vi "Send Command.vi"(8 "error in (no error)":errorcluster, 9 "Thread ID":u16, 10 "Message Queues":T3, 11 "Current Test":T1) -> (0 "error out":errorcluster)   [LabVIEW 2014]
uses:
  support/Message Queue/All Message Queues.ctl
  support/Message Queue/Message Cluster.ctl
  Teszt/Teszt.ctl
  Teszt/Command.ctl
  Message.ctl
  support/Message Queue/Enqueue Message (Single).vi
  support/Message Queue/Message Queue.lvlib
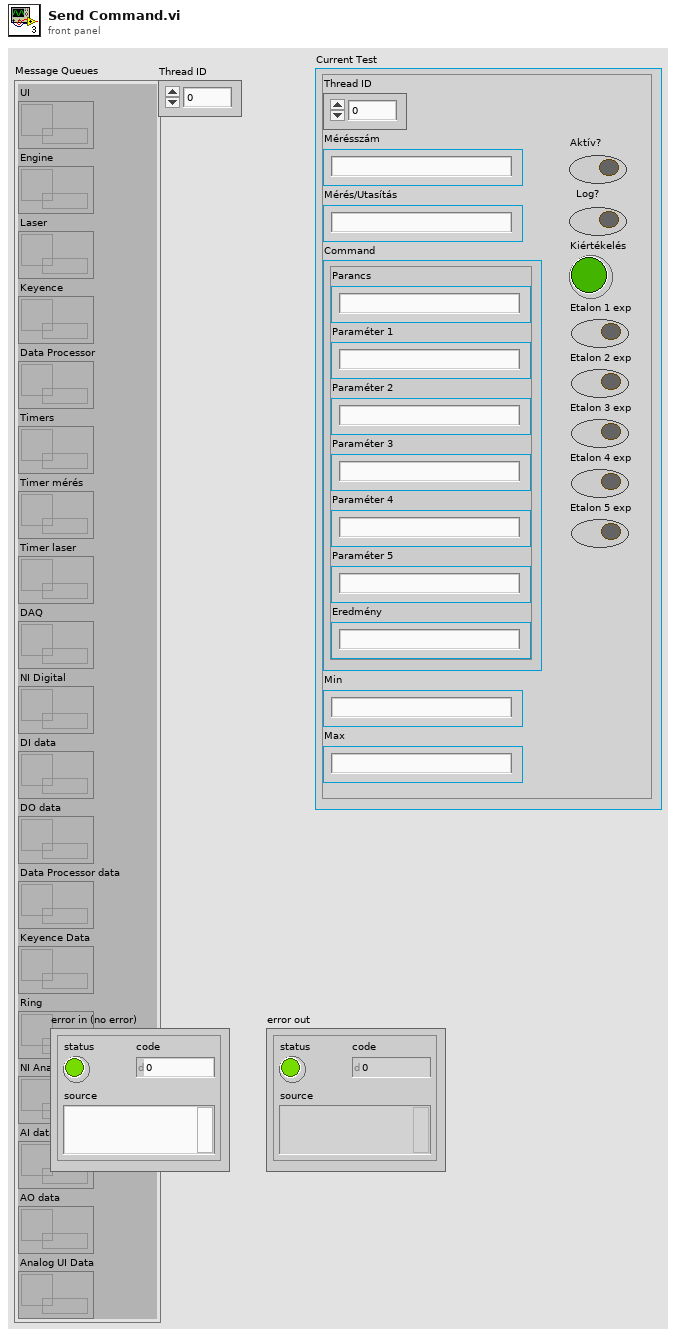
[diagram p1: front panel]
types:
  T1 = typedef "Teszt.ctl" = cluster{"Thread ID":dbl, "Mérésszám":string, "Mérés/Utasítás":string, "Command":T2, "Min":string, "Max":string, "Aktív?":bool, "Log?":bool, "Kiértékelés":bool, "Etalon 1 exp":bool, "Etalon 2 exp":bool, "Etalon 3 exp":bool, "Etalon 4 exp":bool, "Etalon 5 exp":bool}
  T2 = typedef "Command.ctl" = cluster{"Parancs":string, "Paraméter 1":string, "Paraméter 2":string, "Paraméter 3":string, "Paraméter 4":string, "Paraméter 5":string, "Eredmény":string}
  T3 = typedef "Message Queue.lvlib/All Message Queues.ctl" = cluster{"UI":refnum<queue>, "Engine":refnum<queue>, "Laser":refnum<queue>, "Keyence":refnum<queue>, "Data Processor":refnum<queue>, "Timers":refnum<queue>, "Timer mérés":refnum<queue>, "Timer laser":refnum<queue>, "DAQ":refnum<queue>, "NI Digital":refnum<queue>, "DI data":refnum<queue>, "DO data":refnum<queue>, "Data Processor data":refnum<queue>, "Keyence Data":refnum<queue>, "Ring":refnum<queue>, "NI Analog":refnum<queue>, "AI data":refnum<queue>, "AO data":refnum<queue>, "Analog UI Data":refnum<queue>}
  T4 = typedef "Message.ctl" = cluster{"Thread ID":u16, "Callback":string, "Data":variant, "Error":errorcluster}
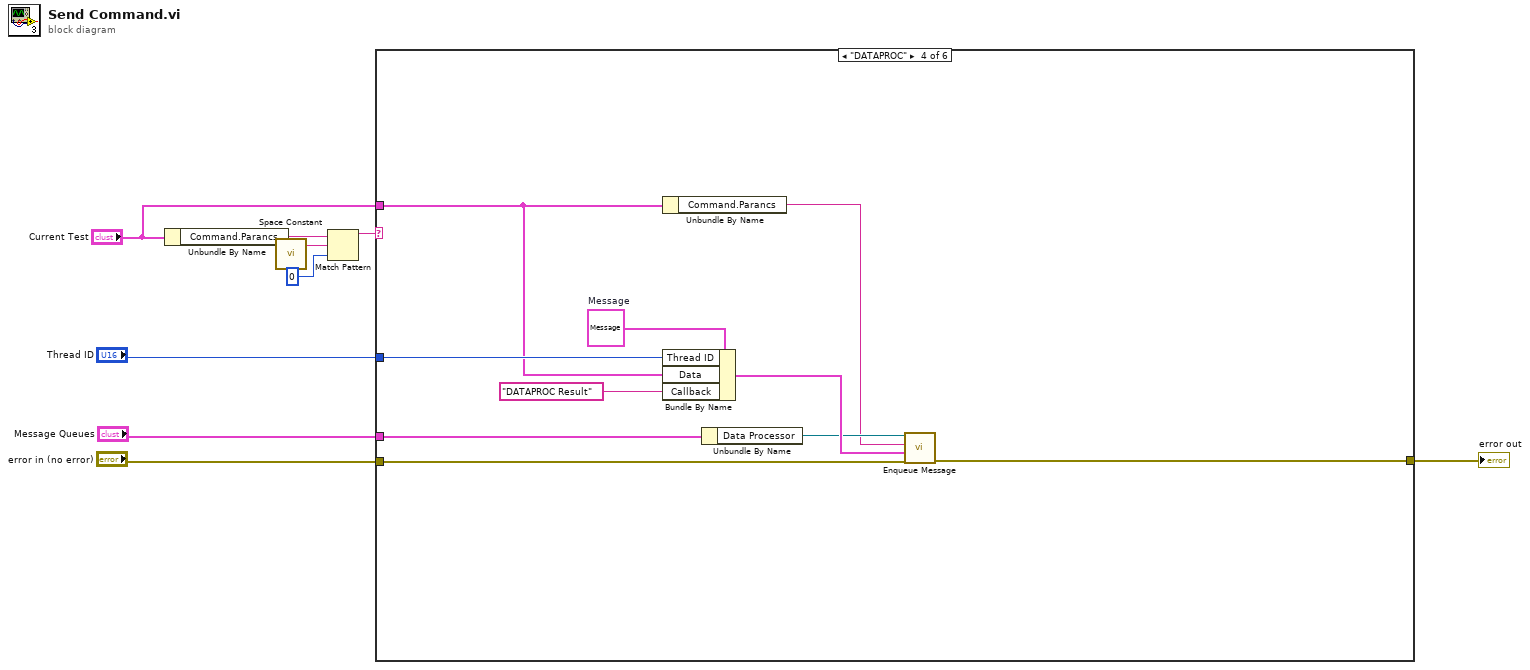
[diagram p0: block diagram]
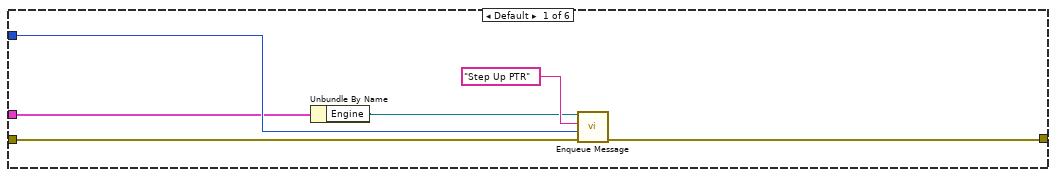
[diagram p2: hidden frame]
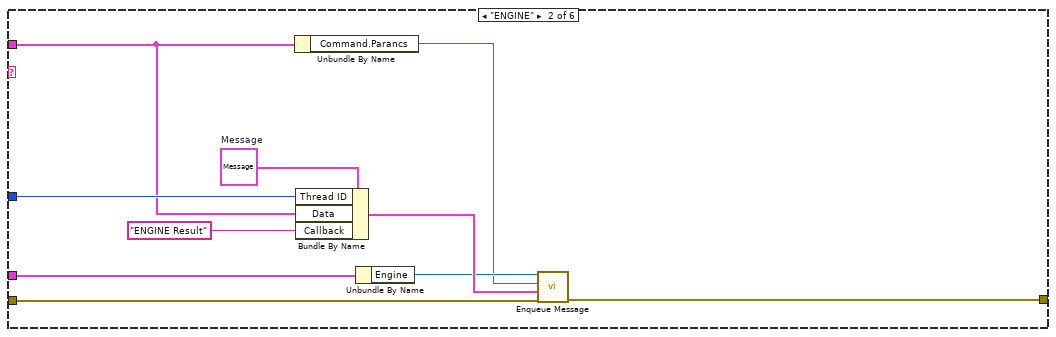
[diagram p3: hidden frame]
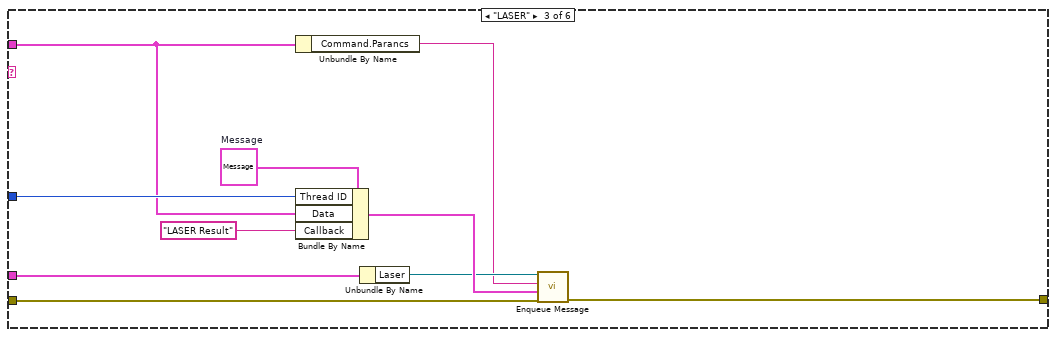
[diagram p4: hidden frame]
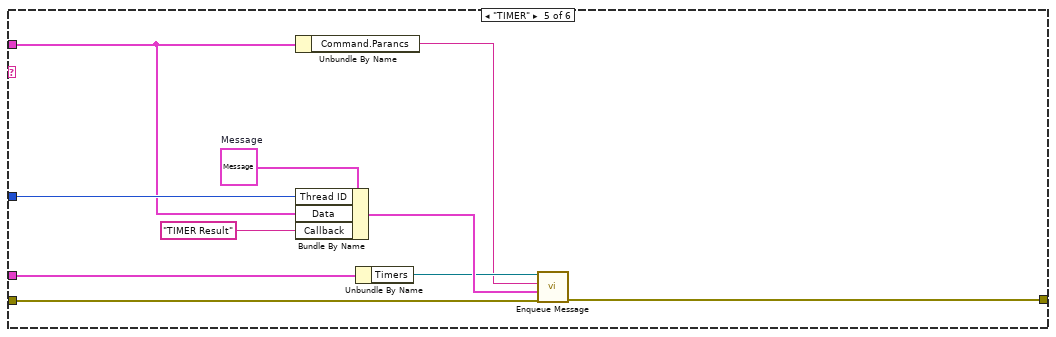
[diagram p5: hidden frame]
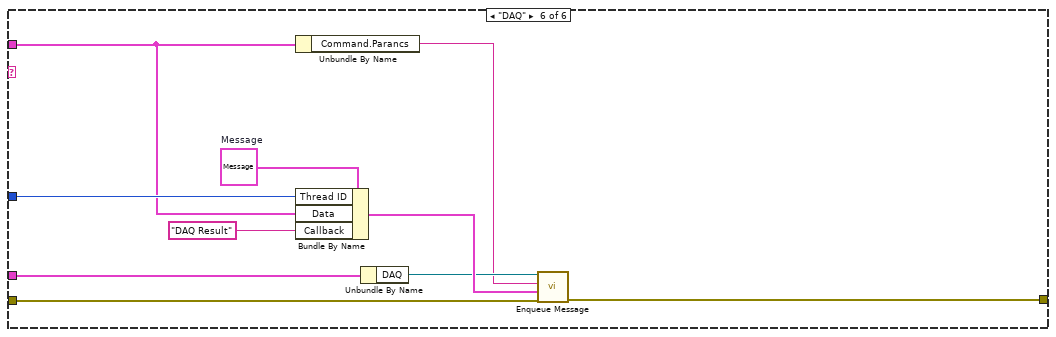
[diagram p6: hidden frame]
diagram:
  n1 = Unbundle By Name("Current Test") -> ("Command.Parancs"=w6:string)
  n2 = call <vilib>:"Space Constant.vi"() -> ("String"=w5:string)
  n3 = Match Pattern(string=w6, regular expression=w5, offset (0)=0) -> (before substring=w3:string)  [unwired: 3 out]
  n4 = case shown="\"DATAPROC\"" w3 {
    tunnel: "Message Queues" -> [w12 w23 w33 w43 w53 w63]
    tunnel: "Thread ID" -> [w13 w22 w32 w42 w52 w62]
    tunnel: "error in (no error)" -> [w14 w21 w31 w41 w51 w61]
    tunnel: "Current Test" -> [_ w17 w27 w37 w47 w57]
    tunnel: [w10 w19 w29 w39 w49 w59] -> w2
    frame Default {
      n5 = Unbundle By Name(w12) -> ("Engine"=w11:refnum<queue>)
      n6 = call-poly "Enqueue Message.vi"("error in (no error)"=w14, "Message Data"=w13, "Message"="Step Up PTR", "Message Queue"=w11) -> ("error out"=w10:errorcluster)  [unwired: 6 in, 1 out]
    }
    frame "ENGINE" {
      w20 = T4 {"Thread ID"=0, "Callback"="", "Data"=variant, "Error"={"status"=FALSE, "code"=0, "source"=""}}  # Message
      n7 = Unbundle By Name(w17) -> ("Command.Parancs"=w16:string)
      n8 = Bundle By Name(cluster=w20, "Thread ID"=w22, "Data"=w17, "Callback"="ENGINE Result") -> (w25:T4)
      n9 = Unbundle By Name(w23) -> ("Engine"=w24:refnum<queue>)
      n10 = call-poly "Enqueue Message.vi"("error in (no error)"=w21, "Message Data"=w25, "Message"=w16, "Message Queue"=w24) -> ("error out"=w19:errorcluster)  [unwired: 6 in, 1 out]
    }
    frame "LASER" {
      w30 = T4 {"Thread ID"=0, "Callback"="", "Data"=variant, "Error"={"status"=FALSE, "code"=0, "source"=""}}  # Message
      n11 = Unbundle By Name(w27) -> ("Command.Parancs"=w26:string)
      n12 = Bundle By Name(cluster=w30, "Thread ID"=w32, "Data"=w27, "Callback"="LASER Result") -> (w35:T4)
      n13 = Unbundle By Name(w33) -> ("Laser"=w34:refnum<queue>)
      n14 = call-poly "Enqueue Message.vi"("error in (no error)"=w31, "Message Data"=w35, "Message"=w26, "Message Queue"=w34) -> ("error out"=w29:errorcluster)  [unwired: 6 in, 1 out]
    }
    frame "DATAPROC" {
      w40 = T4 {"Thread ID"=0, "Callback"="", "Data"=variant, "Error"={"status"=FALSE, "code"=0, "source"=""}}  # Message
      n15 = Unbundle By Name(w37) -> ("Command.Parancs"=w36:string)
      n16 = Bundle By Name(cluster=w40, "Thread ID"=w42, "Data"=w37, "Callback"="DATAPROC Result") -> (w45:T4)
      n17 = Unbundle By Name(w43) -> ("Data Processor"=w44:refnum<queue>)
      n18 = call-poly "Enqueue Message.vi"("error in (no error)"=w41, "Message Data"=w45, "Message"=w36, "Message Queue"=w44) -> ("error out"=w39:errorcluster)  [unwired: 6 in, 1 out]
    }
    frame "TIMER" {
      w50 = T4 {"Thread ID"=0, "Callback"="", "Data"=variant, "Error"={"status"=FALSE, "code"=0, "source"=""}}  # Message
      n19 = Unbundle By Name(w47) -> ("Command.Parancs"=w46:string)
      n20 = Bundle By Name(cluster=w50, "Thread ID"=w52, "Data"=w47, "Callback"="TIMER Result") -> (w55:T4)
      n21 = Unbundle By Name(w53) -> ("Timers"=w54:refnum<queue>)
      n22 = call-poly "Enqueue Message.vi"("error in (no error)"=w51, "Message Data"=w55, "Message"=w46, "Message Queue"=w54) -> ("error out"=w49:errorcluster)  [unwired: 6 in, 1 out]
    }
    frame "DAQ" {
      w60 = T4 {"Thread ID"=0, "Callback"="", "Data"=variant, "Error"={"status"=FALSE, "code"=0, "source"=""}}  # Message
      n23 = Unbundle By Name(w57) -> ("Command.Parancs"=w56:string)
      n24 = Bundle By Name(cluster=w60, "Thread ID"=w62, "Data"=w57, "Callback"="DAQ Result") -> (w65:T4)
      n25 = Unbundle By Name(w63) -> ("DAQ"=w64:refnum<queue>)
      n26 = call-poly "Enqueue Message.vi"("error in (no error)"=w61, "Message Data"=w65, "Message"=w56, "Message Queue"=w64) -> ("error out"=w59:errorcluster)  [unwired: 6 in, 1 out]
    }
  }
  "error out" <- w2
